vi "oa_Buffer and Select Order Waveform.vi"(7 "reset? (F)":bool, 8 "actual samples/rev":dbl format="%.2f", 9 "revolutions":dbl format="%.2f", 10 "start":dbl format="%.2f", 11 "order data":dbl[](array[numeric]) format="%.2f") -> (1 "rev out":dbl format="%.2f", 3 "selected order data":dbl[](array[numeric]) format="%.2f")   [LabVIEW 2017]
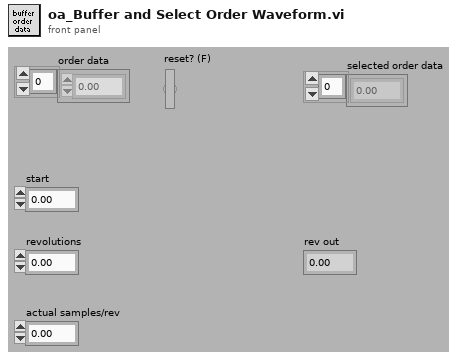
[diagram p1: front panel]
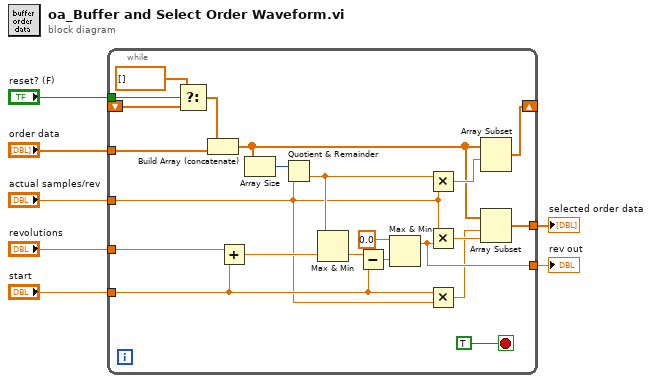
[diagram p0: block diagram]
diagram:
  n1 = while {
    tunnel: "order data" -> [w8]
    shift-right: [w29] -> _
    shift-left: _ -> [w25]
    tunnel: "reset? (F)" -> [w24]
    tunnel: "actual samples/rev" -> [w14]
    tunnel: "start" -> [w15]
    tunnel: "revolutions" -> [w20]
    tunnel: [w13] -> w2
    tunnel: [w11] -> w1
    stop <- TRUE stop-if-true
    n2 = Select(t=dbl[] [], s=w24, f=w25) -> (s? t:f=w28:dbl[])
    n3 = Build Array (concatenate)(w28, w8) -> (w21:dbl[])
    n4 = Add(x=w20, y=w15) -> (x+y=w18:dbl)
    n5 = Array Size(array=w21) -> (size(s)=w27:i32)
    n6 = Quotient & Remainder(x=w27, y=w14) -> (floor(x/y)=w26:dbl)  [unwired: 1 out]
    n7 = Max & Min(x=w26, y=w18) -> (min(x,y)=w19:dbl)  [unwired: 1 out]
    n8 = Subtract(x=w19, y=w15) -> (x-y=w17:dbl)
    n9 = Max & Min(x=0.0, y=w17) -> (max(x,y)=w13:dbl)  [unwired: 1 out]
    n10 = Multiply(x=w26, y=w14) -> (x*y=w22:dbl)
    n11 = Multiply(x=w14, y=w13) -> (x*y=w10:dbl)
    n12 = Multiply(x=w15, y=w14) -> (x*y=w9:dbl)
    n13 = Array Subset(array=w21, index=w22) -> (w29:dbl[])  [unwired: 1 in]
    n14 = Array Subset(array=w21, index=w9, length=w10) -> (w11:dbl[])
  }
  "rev out" <- w2
  "selected order data" <- w1
